vi "Main.vi"() -> ()   [LabVIEW 2026]
doc: "This Continuous Measurement sample project is based on the Queued Message Handler template.\n\nThe Event Handling Loop generates messages based on user interface actions.\n\nThe Message Handling Loop processes messages generated by the Event Handling Loop, or by other messages. There are also Acquisition and Logging message handling loop subVIs, and a chart updating loop."
uses:
  controls/UI State.ctl
  controls/UI Data.ctl
  Settings/Settings.ctl
  Acquisition/Hardware Configuration.ctl
  Acquisition/Signal Type.ctl
  Logging/Logging Configuration.ctl
  support/Message Queue/Enqueue Message (Single).vi
  support/Message Queue/Enqueue Message (Array).vi
  <vilib>/Utility/error.llb/Error Cluster From Error Code.vi
  <vilib>/ErrorRing/Error Ring.xnode
  Acquisition/Acquisition.lvlib
  Logging/Logging.lvlib
  Settings/Settings.lvlib
  support/User Event - Stop/User Event - Stop.lvlib
  support/Message Queue/Message Queue.lvlib
  Settings/Settings Dialog.vi
panel:
  out "Hardware Configuration.HW Refnum <Replace Me>":string
  out "Hardware Configuration.Signal Type <Replace Me>":T1
  out "Data":waveform(dbl)[](graph)
  in  "Settings":bool
  in  "Start":bool
  in  "Stop":bool
  out "Status":string
  in  "Exit":bool
  # "Continuous Measurement Data Logger"
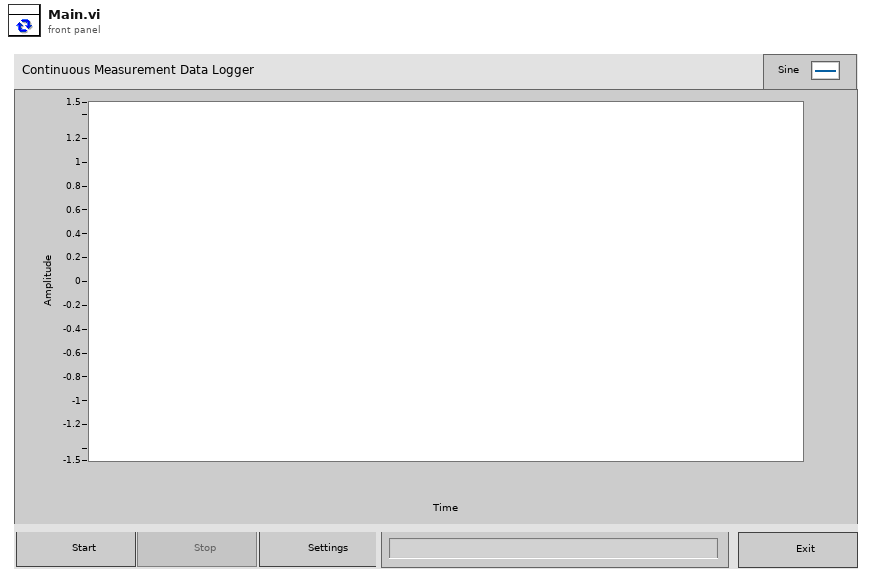
[diagram p1: front panel]
types:
  T1 = typedef "Acquisition.lvlib/Signal Type.ctl" = enum16{"Sine Wave", "Square with Noise"}
  T2 = typedef "UI State.ctl" = enum16{"Idle", "Acquiring and Logging", "Waiting for Exit", "Waiting for Exit (Acq Stopped)", "Waiting for Exit (Log Stopped)", "Waiting for Stop", "Waiting for Stop (Acq Stopped)", "Waiting for Stop (Log Stopped)"}
  T3 = typedef "UI Data.ctl" = cluster{"Start Ref":refnum<vi>, "Stop Ref":refnum<vi>, "Settings Ref":refnum<vi>, "Exit Ref":refnum<vi>, "Status Ref":refnum<vi>, "Data Ref":refnum<vi>}
  T4 = typedef "Settings.lvlib/Settings.ctl" = cluster{"Hardware Configuration":T5, "Logging Configuration":T6}
  T5 = typedef "Acquisition.lvlib/Hardware Configuration.ctl" = cluster{"HW Refnum <Replace Me>":string, "Signal Type <Replace Me>":T1}
  T6 = typedef "Logging.lvlib/Logging Configuration.ctl" = cluster{"Log File Base Path":path, "TDMS File Reference":refnum<k34>}
  T7 = typedef "Message Queue.lvlib/All Message Queues.ctl" = cluster{"UI":refnum<queue>, "Acquisition":refnum<queue>, "Logging":refnum<queue>}
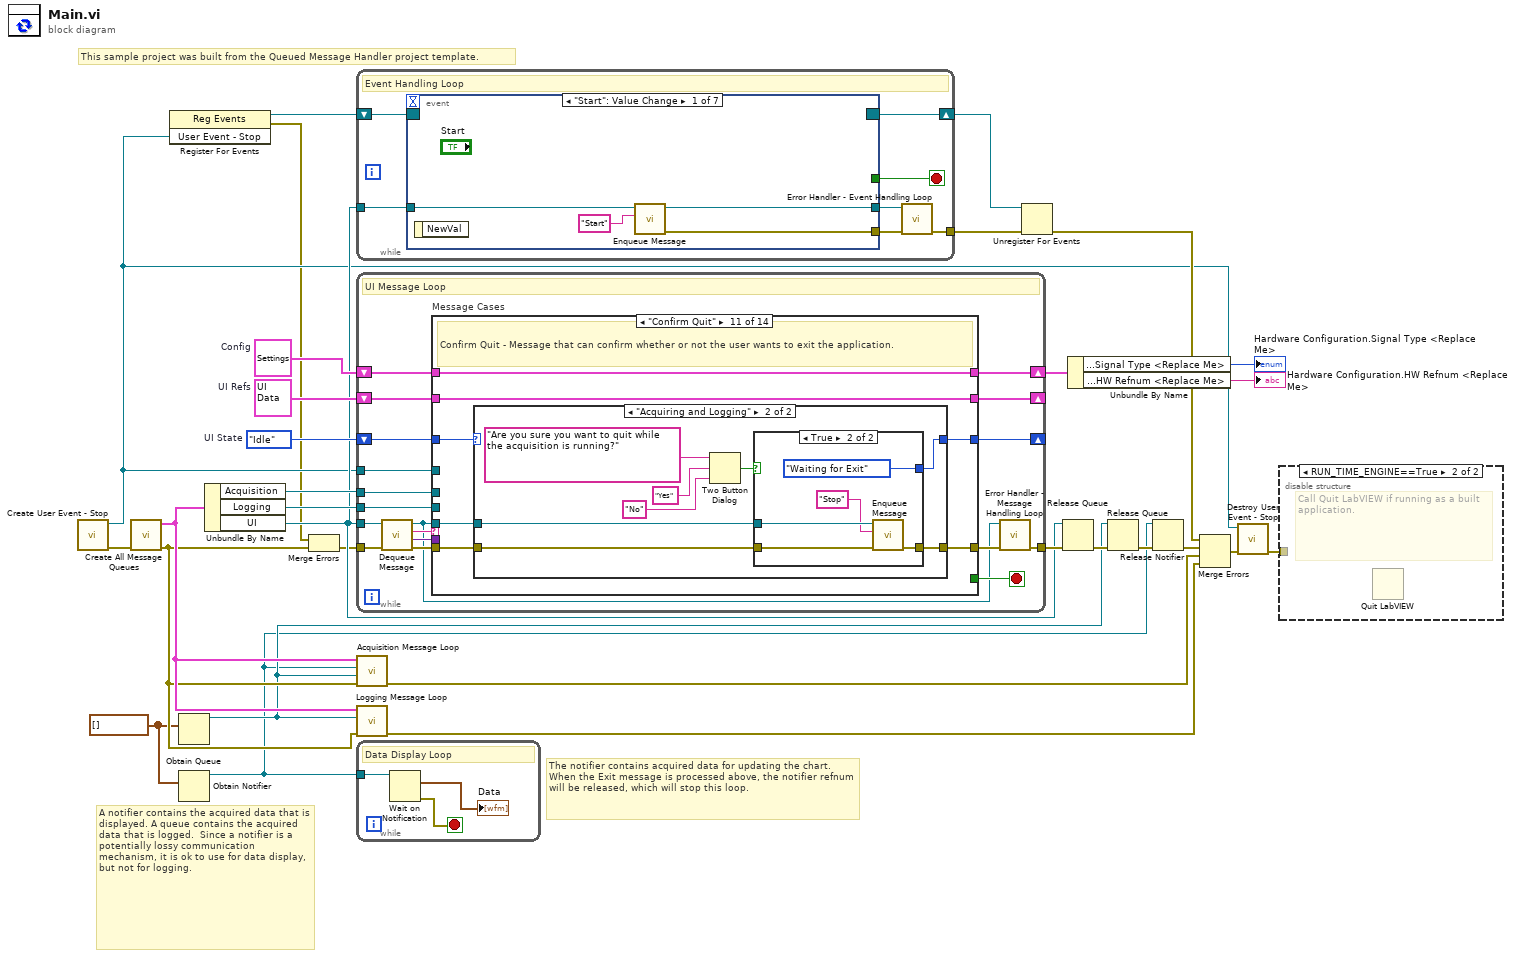
[diagram p0: block diagram]
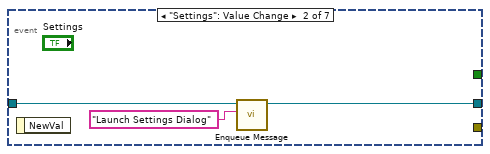
[diagram p3: hidden frame]
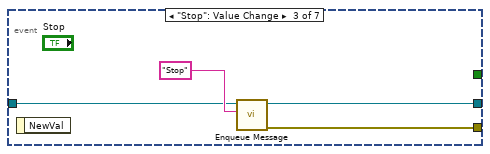
[diagram p4: hidden frame]
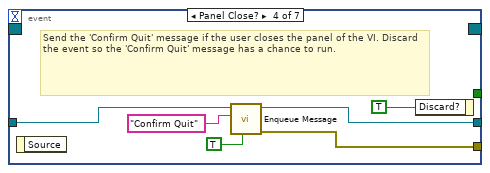
[diagram p5: hidden frame]
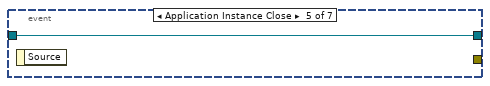
[diagram p6: hidden frame]
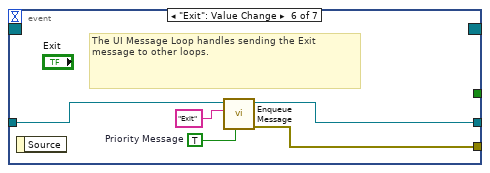
[diagram p7: hidden frame]
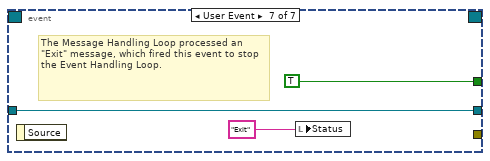
[diagram p8: hidden frame]
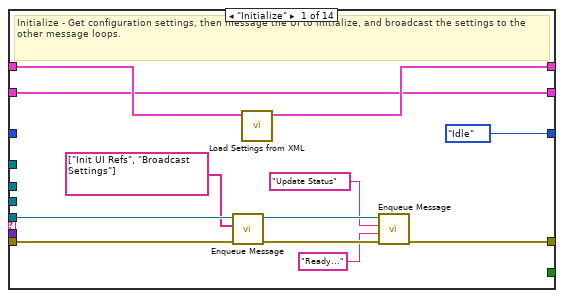
[diagram p9: hidden frame]
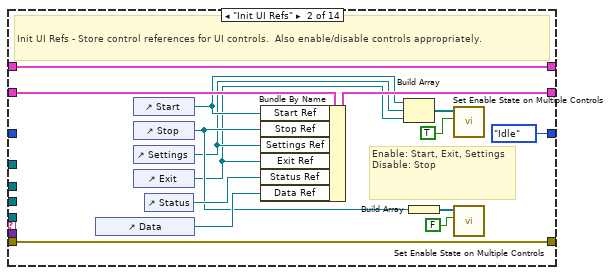
[diagram p10: hidden frame]
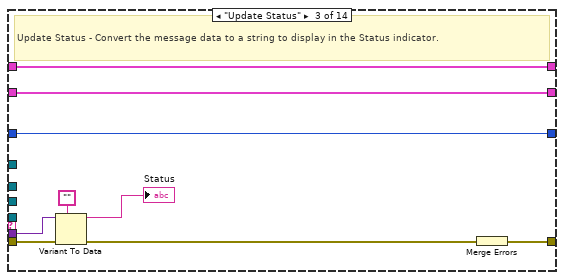
[diagram p11: hidden frame]
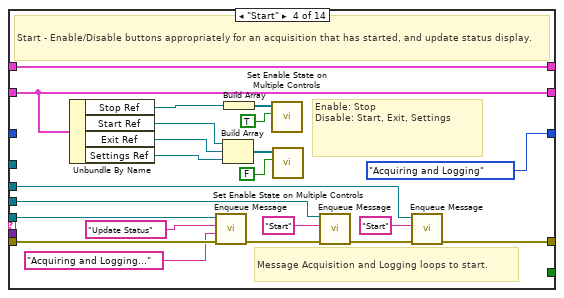
[diagram p12: hidden frame]
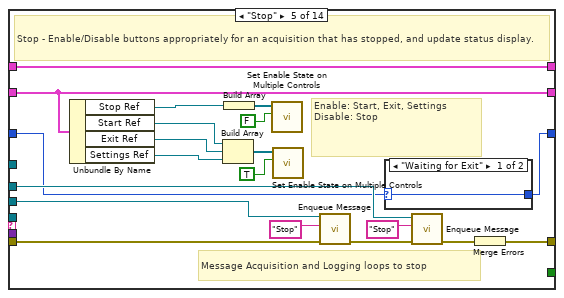
[diagram p13: hidden frame]
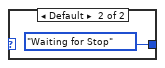
[diagram p14: hidden frame]
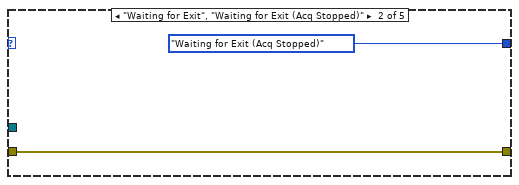
[diagram p16: hidden frame]
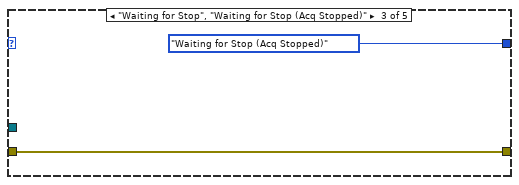
[diagram p17: hidden frame]
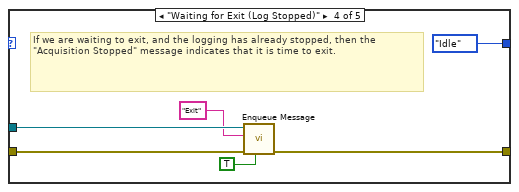
[diagram p18: hidden frame]
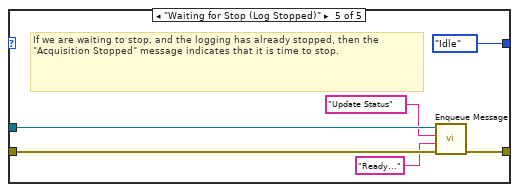
[diagram p19: hidden frame]
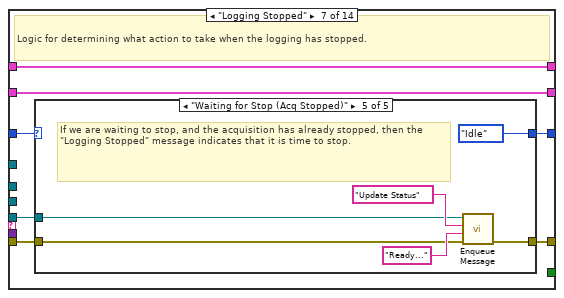
[diagram p20: hidden frame]
diagram:
  w17 = UI_State."Idle"  # UI State
  w8 = waveform(dbl)[] []
  w20 = T3 {"Start Ref"=refnum, "Stop Ref"=refnum, "Settings Ref"=refnum, "Exit Ref"=refnum, "Status Ref"=refnum, "Data Ref"=refnum}  # UI Refs
  w23 = T4 {"Hardware Configuration"={"HW Refnum <Replace Me>"="", "Signal Type <Replace Me>"=enum."Sine Wave"}, "Logging Configuration"={"Log File Base Path"=path "", "TDMS File Reference"=refnum}}  # Config
  # "This sample project was built from the Queued Message Handler project template."
  # "A notifier contains the acquired data that is displayed. A queue contains the acquired data that is logged.  Since a notifier is a potentially lossy communication mechanism, it is ok to use for data display, but not for logging."
  # "The notifier contains acquired data for updating the chart. When the Exit message is processed above, the notifier refnum will be released, which will stop this loop."
  n1 = call "Create User Event - Stop.vi"() -> ("error out"=w27:errorcluster, "User Event - Stop"=w6:refnum<user-event>)  [unwired: 10 in]
  n2 = call "Create All Message Queues.vi"("error in (no error)"=w27) -> ("error out"=w24:errorcluster, "Message Queues out"=w26:T7)  [unwired: 9 in]
  n3 = register-events(w6) -> (reference out=w7:refnum<event-registration>, error out=w4:errorcluster)  [unwired: 2 in]
  n4 = Obtain Queue(element data type=w8) -> (queue out=w10:refnum<queue>)  [unwired: 4 in, 2 out]
  n5 = Obtain Notifier(notification data type=w8) -> (notifier out=w9:refnum<notifier>)  [unwired: 3 in, 2 out]
  n6 = Unbundle By Name(w26) -> ("Acquisition"=w19:refnum<queue>, "Logging"=w18:refnum<queue>, "UI"=w15:refnum<queue>)
  n7 = Merge Errors(w4, w24) -> (w5:errorcluster)
  n8 = while {
    tunnel: w15 -> [w36]
    tunnel: [w33] -> w29
    shift-right: [w35] -> w21
    shift-left: w7 -> [w37]
    stop <- w34 stop-if-true
    # "Event Handling Loop"
    n9 = event shown="[0] \"Start\": Value Change" {
      selector: w37 -> [_ _ _ _ _ _ _]
      dyn-events: [_ _ _ _ _ _ _] -> w35
      timeout: _ -> [_ _ _ _ _ _ _]
      tunnel: [_ _ _ _ _ _ TRUE ("Discard?")] -> w34
      tunnel: w36 -> [w41 w43 w47 w52 w55 w57 w61]
      tunnel: [w39 _ w46 w50 _ w60 _] -> w32
      tunnel: [w38 w42 w45 w51 w55 w56 w61] -> w31
      event "Start": Value Change {
        n10 = event-data() -> ()  [unwired: 1 in, 1 out]
        n11 = call-poly "Enqueue Message.vi"("Message"="Start", "Message Queue"=w41) -> ("error out"=w39:errorcluster, "dup Message Queue"=w38:refnum<queue>)  [unwired: 8 in]
      }
      event "Settings": Value Change {
        n12 = event-data() -> ()  [unwired: 1 in, 1 out]
        n13 = call-poly "Enqueue Message.vi"("Message"="Launch Settings Dialog", "Message Queue"=w43) -> ("dup Message Queue"=w42:refnum<queue>)  [unwired: 8 in, 1 out]
      }
      event "Stop": Value Change {
        n14 = event-data() -> ()  [unwired: 1 in, 1 out]
        n15 = call-poly "Enqueue Message.vi"("Message"="Stop", "Message Queue"=w47) -> ("error out"=w46:errorcluster, "dup Message Queue"=w45:refnum<queue>)  [unwired: 8 in]
      }
      event Panel Close? {
        # "Send the 'Confirm Quit' message if the user closes the panel of the VI. Discard the event so the 'Confirm Quit' message has a chance to run."
        n16 = event-data() -> ()  [unwired: 1 in, 1 out]
        n17 = call-poly "Enqueue Message.vi"("Priority Message? (F)"=TRUE, "Message"="Confirm Quit", "Message Queue"=w52) -> ("error out"=w50:errorcluster, "dup Message Queue"=w51:refnum<queue>)  [unwired: 7 in]
        n18 = event-data("Discard?"=TRUE) -> ()  [unwired: 1 in, 1 out]
      }
      event Application Instance Close {
        n19 = event-data() -> ()  [unwired: 1 in, 1 out]
      }
      event "Exit": Value Change {
        w58 = TRUE  # Priority Message
        # "The UI Message Loop handles sending the Exit message to other loops."
        n20 = event-data() -> ()  [unwired: 1 in, 1 out]
        n21 = call-poly "Enqueue Message.vi"("Priority Message? (F)"=w58, "Message"="Exit", "Message Queue"=w57) -> ("error out"=w60:errorcluster, "dup Message Queue"=w56:refnum<queue>)  [unwired: 7 in]
      }
      event User Event {
        # "The Message Handling Loop processed an \"Exit\" message, which fired this event to stop the Event Handling Loop."
        n22 = event-data() -> ()  [unwired: 1 in, 1 out]
        n23 = local write "Status"("Exit" ("Exit String")) -> ()
      }
    }
    n24 = call "Error Handler - Event Handling Loop.vi"("error in (no error)"=w32, "Message Queue"=w31) -> ("dup error in"=w33:errorcluster)  [unwired: 8 in, 1 out]
  }
  n25 = while {
    tunnel: w15 -> [w75]
    tunnel: w6 -> [w80]
    shift-right: [w74] -> w3
    shift-left: w23 -> [w73]
    shift-right: [w71] -> _
    shift-left: w20 -> [w72]
    tunnel: w19 -> [w70]
    tunnel: w18 -> [w69]
    shift-right: [w64] -> _
    shift-left: w17 -> [w65]
    tunnel: w5 -> [w79]
    tunnel: [w68] -> w30
    stop <- w81 stop-if-true
    # "UI Message Loop"
    n26 = call "Dequeue Message.vi"("error in (no error)"=w79, "Message Queue"=w75) -> ("error out"=w78:errorcluster, "Message Data"=w76:variant, "Message"=w77:string, "dup Message Queue"=w66:refnum<queue>)  [unwired: 6 in]
    n27 = case "Message Cases" shown="\"Confirm Quit\"" w77 {
      selector: w77 -> [_ _ _ _ _ _ _ _ _ _ _ _ _ w297]
      tunnel: w66 -> [w85 _ _ w139 _ w164 w189 _ w229 _ w250 _ _ _]
      tunnel: w78 -> [w84 w108 w116 w138 w158 w165 w190 w217 w231 w238 w249 w278 w295 _]
      tunnel: [w89 w108 w117 w121 w159 w162 w187 w223 w224 w241 w248 w288 w294 w296] -> w67
      tunnel: [_ _ _ _ _ _ _ _ _ _ _ TRUE _ _] -> w81
      tunnel: w76 -> [_ _ w115 _ _ _ _ _ _ w242 _ w276 _ _]
      tunnel: w80 -> [_ _ _ _ _ _ _ _ _ _ _ w289 _ _]
      tunnel: [w92 w107 w111 w137 w157 w168 w193 w221 w228 w246 w253 w287 w293 w300] -> w74
      tunnel: w73 -> [w93 w107 w111 w137 w157 w168 w193 w221 w232 w246 w253 w287 w293 w300]
      tunnel: w72 -> [w86 w106 w110 w134 w156 w167 w192 w215 w226 w245 w252 w286 w292 w299]
      tunnel: [w86 w103 w110 w134 w156 w167 w192 w215 w226 w245 w252 w286 w292 w299] -> w71
      tunnel: w70 -> [_ _ _ w120 w143 _ _ w214 _ _ _ w285 _ _]
      tunnel: w69 -> [_ _ _ w123 w146 _ _ w213 _ _ _ w284 _ _]
      tunnel: w65 -> [_ _ w109 _ w140 w166 w191 w212 w225 w240 w251 _ w291 w298]
      tunnel: [UI_State."Idle" ("UI State") UI_State."Idle" ("UI State") w109 UI_State."Acquiring and Logging" ("UI State") w141 w163 w188 w212 w225 w240 w247 UI_State."Idle" ("UI State") w291 w298] -> w64
      frame "Initialize" {
        # "Initialize - Get configuration settings, then message the UI to initialize, and broadcast the settings to the other message loops."
        n28 = call-poly "Enqueue Message.vi"("error in (no error)"=w84, "Message Array"=string[] ["Init UI Refs", "Broadcast Settings"], "Message Queue"=w85) -> ("error out"=w91:errorcluster, "dup Message Queue"=w90:refnum<queue>)  [unwired: 7 in]
        n29 = call "Load Settings from XML.vi"("Settings in"=w93) -> ("Settings out"=w92:T4)  [unwired: 9 in, 1 out]
        n30 = call-poly "Enqueue Message.vi"("error in (no error)"=w91, "Message Data"="Ready..." ("Ready..."), "Message"="Update Status", "Message Queue"=w90) -> ("error out"=w89:errorcluster)  [unwired: 6 in, 1 out]
      }
      frame "Init UI Refs" {
        # "Enable: Start, Exit, Settings\nDisable: Stop"
        # "Init UI Refs - Store control references for UI controls.  Also enable/disable controls appropriately."
        n31 = control-ref of="Data"() -> (w104:refnum<vi>)
        n32 = control-ref of="Start"() -> (w97:refnum<vi>)
        n33 = control-ref of="Stop"() -> (w98:refnum<vi>)
        n34 = control-ref of="Settings"() -> (w96:refnum<vi>)
        n35 = control-ref of="Exit"() -> (w95:refnum<vi>)
        n36 = control-ref of="Status"() -> (w105:refnum<vi>)
        n37 = Bundle By Name(cluster=w106, "Start Ref"=w97, "Stop Ref"=w98, "Settings Ref"=w96, "Exit Ref"=w95, "Status Ref"=w105, "Data Ref"=w104) -> (w103:T3)
        n38 = Build Array(w97, w96, w95) -> (w101:refnum<vi>[])
        n39 = Build Array(w98) -> (w100:refnum<vi>[])
        n40 = call "Set Enable State on Multiple Controls.vi"("Enable?"=TRUE, "Controls"=w101) -> ()  [unwired: 10 in]
        n41 = call "Set Enable State on Multiple Controls.vi"("Enable?"=FALSE, "Controls"=w100) -> ()  [unwired: 10 in]
      }
      frame "Update Status" {
        # "Update Status - Convert the message data to a string to display in the Status indicator."
        n42 = Variant To Data(error in=w116, type="", Variant=w115) -> (data=→"Status":string, error out=w113:errorcluster)
        n43 = Merge Errors(w113) -> (w117:errorcluster)
      }
      frame "Start" {
        # "Message Acquisition and Logging loops to start."
        # "Enable: Stop\nDisable: Start, Exit, Settings"
        # "Start - Enable/Disable buttons appropriately for an acquisition that has started, and update status display."
        n44 = Unbundle By Name(w134) -> ("Stop Ref"=w129:refnum<vi>, "Start Ref"=w128:refnum<vi>, "Exit Ref"=w127:refnum<vi>, "Settings Ref"=w126:refnum<vi>)
        n45 = call-poly "Enqueue Message.vi"("error in (no error)"=w138, "Message Data"="Acquiring and Logging..." ("Acquiring and Logging..."), "Message"="Update Status", "Message Queue"=w139) -> ("error out"=w125:errorcluster)  [unwired: 6 in, 1 out]
        n46 = Build Array(w128, w127, w126) -> (w132:refnum<vi>[])
        n47 = Build Array(w129) -> (w131:refnum<vi>[])
        n48 = call "Set Enable State on Multiple Controls.vi"("Enable?"=TRUE, "Controls"=w131) -> ()  [unwired: 10 in]
        n49 = call "Set Enable State on Multiple Controls.vi"("Enable?"=FALSE, "Controls"=w132) -> ()  [unwired: 10 in]
        n50 = call-poly "Enqueue Message.vi"("error in (no error)"=w125, "Message"="Start", "Message Queue"=w123) -> ("error out"=w122:errorcluster)  [unwired: 7 in, 1 out]
        n51 = call-poly "Enqueue Message.vi"("error in (no error)"=w122, "Message"="Start", "Message Queue"=w120) -> ("error out"=w121:errorcluster)  [unwired: 7 in, 1 out]
      }
      frame "Stop" {
        # "Message Acquisition and Logging loops to stop"
        # "Enable: Start, Exit, Settings\nDisable: Stop"
        # "Stop - Enable/Disable buttons appropriately for an acquisition that has stopped, and update status display."
        n52 = Unbundle By Name(w156) -> ("Stop Ref"=w151:refnum<vi>, "Start Ref"=w150:refnum<vi>, "Exit Ref"=w149:refnum<vi>, "Settings Ref"=w148:refnum<vi>)
        n53 = Build Array(w150, w149, w148) -> (w154:refnum<vi>[])
        n54 = Build Array(w151) -> (w153:refnum<vi>[])
        n55 = call "Set Enable State on Multiple Controls.vi"("Enable?"=FALSE, "Controls"=w153) -> ()  [unwired: 10 in]
        n56 = call "Set Enable State on Multiple Controls.vi"("Enable?"=TRUE, "Controls"=w154) -> ()  [unwired: 10 in]
        n57 = call-poly "Enqueue Message.vi"("error in (no error)"=w158, "Message"="Stop", "Message Queue"=w146) -> ("error out"=w145:errorcluster)  [unwired: 7 in, 1 out]
        n58 = case shown="\"Waiting for Exit\"" w140 {
          selector: w140 -> [w160 _]
          tunnel: [w160 UI_State."Waiting for Stop" ("UI State")] -> w141
          frame "Waiting for Exit" {
          }
          frame Default {
          }
        }
        n59 = call-poly "Enqueue Message.vi"("error in (no error)"=w145, "Message"="Stop", "Message Queue"=w143) -> ("error out"=w144:errorcluster)  [unwired: 7 in, 1 out]
        n60 = Merge Errors(w144) -> (w159:errorcluster)
      }
      frame "Acquisition Stopped" {
        # "Logic for determining what action to take when the acquisition has stopped."
        n61 = case shown="Default" w166 {
          selector: w166 -> [w170 _ _ _ _]
          tunnel: w165 -> [w169 w172 w174 w180 w186]
          tunnel: w164 -> [_ _ _ w178 w183]
          tunnel: [w170 UI_State."Waiting for Exit (Acq Stopped)" ("UI State") UI_State."Waiting for Stop (Acq Stopped)" ("UI State") UI_State."Idle" ("UI State") UI_State."Idle" ("UI State")] -> w163
          tunnel: [w169 w172 w174 w179 w184] -> w162
          frame Default {
          }
          frame "Waiting for Exit", "Waiting for Exit (Acq Stopped)" {
          }
          frame "Waiting for Stop", "Waiting for Stop (Acq Stopped)" {
          }
          frame "Waiting for Exit (Log Stopped)" {
            # "If we are waiting to exit, and the logging has already stopped, then the \"Acquisition Stopped\" message indicates that it is time to exit."
            n62 = call-poly "Enqueue Message.vi"("Priority Message? (F)"=TRUE, "error in (no error)"=w180, "Message"="Exit", "Message Queue"=w178) -> ("error out"=w179:errorcluster)  [unwired: 6 in, 1 out]
          }
          frame "Waiting for Stop (Log Stopped)" {
            # "If we are waiting to stop, and the logging has already stopped, then the \"Acquisition Stopped\" message indicates that it is time to stop."
            n63 = call-poly "Enqueue Message.vi"("error in (no error)"=w186, "Message Data"="Ready..." ("Ready..."), "Message"="Update Status", "Message Queue"=w183) -> ("error out"=w184:errorcluster)  [unwired: 6 in, 1 out]
          }
        }
      }
      frame "Logging Stopped" {
        # "Logic for determining what action to take when the logging has stopped."
        n64 = case shown="\"Waiting for Stop (Acq Stopped)\"" w191 {
          selector: w191 -> [w195 _ _ _ _]
          tunnel: w190 -> [w194 w197 w199 w205 w208]
          tunnel: w189 -> [_ _ _ w203 w207]
          tunnel: [w195 UI_State."Waiting for Exit (Log Stopped)" ("UI State") UI_State."Waiting for Stop (Log Stopped)" ("UI State") UI_State."Idle" ("UI State") UI_State."Idle" ("UI State")] -> w188
          tunnel: [w194 w197 w199 w204 w206] -> w187
          frame Default {
          }
          frame "Waiting for Exit", "Waiting for Exit (Log Stopped)" {
          }
          frame "Waiting for Stop", "Waiting for Stop (Log Stopped)" {
          }
          frame "Waiting for Exit (Acq Stopped)" {
            # "If we are waiting to exit, and the acquisition has already stopped, then the \"Logging Stopped\" message indicates that it is time to exit."
            n65 = call-poly "Enqueue Message.vi"("Priority Message? (F)"=TRUE, "error in (no error)"=w205, "Message"="Exit", "Message Queue"=w203) -> ("error out"=w204:errorcluster)  [unwired: 6 in, 1 out]
          }
          frame "Waiting for Stop (Acq Stopped)" {
            # "If we are waiting to stop, and the acquisition has already stopped, then the \"Logging Stopped\" message indicates that it is time to stop."
            n66 = call-poly "Enqueue Message.vi"("error in (no error)"=w208, "Message Data"="Ready..." ("Ready..."), "Message"="Update Status", "Message Queue"=w207) -> ("error out"=w206:errorcluster)  [unwired: 6 in, 1 out]
          }
        }
      }
      frame "Broadcast settings" {
        w216 = "Update Settings" ("Message")
        # "Broadcast settings - Send the 'Update Settings' message to the Logging and Acquisition message loops."
        n67 = Unbundle By Name(w221) -> ("Hardware Configuration"=w220:T5, "Logging Configuration"=w219:T6)
        n68 = call-poly "Enqueue Message.vi"("Message Data"=w220, "Message"=w216, "Message Queue"=w214) -> ("error out"=w222:errorcluster)  [unwired: 7 in, 1 out]
        n69 = call-poly "Enqueue Message.vi"("error in (no error)"=w222, "Message Data"=w219, "Message"=w216, "Message Queue"=w213) -> ("error out"=w218:errorcluster)  [unwired: 6 in, 1 out]
        n70 = Merge Errors(w218, w217) -> (w223:errorcluster)
      }
      frame "Launch Settings Dialog" {
        # "Launch Settings Dialog - Launch the Settings Dialog when the user clicks the 'Settings' button."
        n71 = call-by-ref "?"("error in (no error)"=w231, "Settings in"=w232) -> ("error out"=w227:errorcluster, "Cancelled?"=w230:bool, "Settings out"=w228:T4)  [unwired: 8 in, 3 out]
        n72 = case shown="False" w230 {
          tunnel: w229 -> [w236 _]
          tunnel: w227 -> [w235 w237]
          tunnel: [w234 w237] -> w224
          frame False {
            n73 = call-poly "Enqueue Message.vi"("error in (no error)"=w235, "Message"="Broadcast Settings", "Message Queue"=w236) -> ("error out"=w234:errorcluster)  [unwired: 7 in, 1 out]
          }
          frame True {
          }
        }
      }
      frame "Error" {
        # "Error - Display an error dialog. This message is sent by the \"Error Handler\" VIs at the end of other loops in this application."
        n74 = Variant To Data(error in=w238, type=errorcluster {"status"=FALSE, "code"=0, "source"=""} ("error constant"), Variant=w242) -> (data=w239:errorcluster, error out=w243:errorcluster)
        n75 = call <vilib>:"Simple Error Handler.vi"("error in (no error)"=w239) -> ()  [unwired: 4 in, 5 out]
        n76 = Merge Errors(w243) -> (w241:errorcluster)
      }
      frame "Confirm Quit" {
        # "Confirm Quit - Message that can confirm whether or not the user wants to exit the application."
        n77 = case shown="\"Acquiring and Logging\"" w251 {
          tunnel: w250 -> [w259 w263]
          tunnel: w249 -> [w258 w262]
          tunnel: [w257 w261] -> w248
          tunnel: [UI_State."Idle" ("UI State") w260] -> w247
          frame Default {
            # "If 'Confirm Quit' comes in while the system is idle, there is no need for a confirmation message."
            n78 = call-poly "Enqueue Message.vi"("Priority Message? (F)"=TRUE, "error in (no error)"=w258, "Message"="Exit", "Message Queue"=w259) -> ("error out"=w257:errorcluster)  [unwired: 6 in, 1 out]
          }
          frame "Acquiring and Logging" {
            n79 = Two Button Dialog(message="Are you sure you want to quit while the acquisition is running?" ("Confirm Quit Message"), 1:"No" ("No"), 2:"Yes" ("Yes")) -> (T button?=w264:bool)
            n80 = case shown="True" w264 {
              tunnel: w263 -> [_ w273]
              tunnel: w262 -> [w269 w274]
              tunnel: [w269 w272] -> w261
              tunnel: [UI_State."Acquiring and Logging" ("UI State") UI_State."Waiting for Exit" ("UI State")] -> w260
              frame False {
                # "User did not want to quit."
              }
              frame True {
                n81 = call-poly "Enqueue Message.vi"("error in (no error)"=w274, "Message"="Stop", "Message Queue"=w273) -> ("error out"=w272:errorcluster)  [unwired: 7 in, 1 out]
              }
            }
          }
        }
      }
      frame "Exit" {
        w280 = TRUE ("Priority Message? (F)")
        w281 = "Exit" ("Message")
        # "Popup an error dialog if 'Exit' was called as a result of an error."
        # "Stop the VI"
        # "Exit - Send Exit messages to the Acquisition and Logging loops, and fire the user event to stop the Event Handling Loop."
        n82 = Variant To Data(type=errorcluster {"status"=FALSE, "code"=0, "source"=""} ("error constant"), Variant=w276) -> (data=w275:errorcluster)  [unwired: 1 in, 1 out]
        n83 = call <vilib>:"Simple Error Handler.vi"("error in (no error)"=w275) -> ()  [unwired: 4 in, 5 out]
        n84 = call-poly "Enqueue Message.vi"("Priority Message? (F)"=w280, "error in (no error)"=w278, "Message"=w281, "Message Queue"=w285) -> ("error out"=w282:errorcluster)  [unwired: 6 in, 1 out]
        n85 = call-poly "Enqueue Message.vi"("Priority Message? (F)"=w280, "error in (no error)"=w282, "Message"=w281, "Message Queue"=w284) -> ("error out"=w279:errorcluster)  [unwired: 6 in, 1 out]
        n86 = call "Fire User Event - Stop.vi"("error in (no error)"=w279, "User Event - Stop"=w289) -> ("error out"=w288:errorcluster)  [unwired: 9 in]
      }
      frame "---Copy This Frame---" {
        # "Duplicate this frame when creating new messages.  Change this comment in the duplicated frame to describe this message."
        n87 = Merge Errors(w295) -> (w294:errorcluster)
      }
      frame Default {
        # "'Default' case only runs if there is a message that isn't defined in any of the other cases.  Output a programming error."
        n88 = xnode "Error Ring"("parameter 0"=w297) -> ("error out"=w296:errorcluster)
      }
    }
    n89 = call "Error Handler - Message Handling Loop.vi"("error in (no error)"=w67, "Message Queue"=w66) -> ("dup error in"=w68:errorcluster)  [unwired: 8 in, 1 out]
  }
  n90 = call "Acquisition Message Loop.vi"("error in (no error)"=w24, "Data Queue"=w10, "Data Notifier"=w9, "Message Queues"=w26) -> ("error out"=w28:errorcluster)  [unwired: 7 in]
  n91 = call "Logging Message Loop.vi"("error in (no error)"=w24, "Data Queue"=w10, "Message Queues"=w26) -> ("error out"=w25:errorcluster)  [unwired: 8 in]
  n92 = while "Data Display Loop" {
    tunnel: w9 -> [w310]
    stop <- w308 stop-if-true
    # "Data Display Loop"
    n93 = Wait on Notification(notifier=w310) -> (notification=→"Data":waveform(dbl)[], error out=w308:errorcluster)  [unwired: 3 in, 2 out]
  }
  n94 = Unregister For Events(event registration refnum=w21, error in=w29) -> (error out=w22:errorcluster)
  n95 = Release Queue(queue=w15, error in (no error)=w30) -> (error out=w13:errorcluster)  [unwired: 1 in, 2 out]
  n96 = Unbundle By Name(w3) -> ("Hardware Configuration.Signal Type <Replace Me>"=→"Hardware Configuration.Signal Type <Replace Me>":T1, "Hardware Configuration.HW Refnum <Replace Me>"=→"Hardware Configuration.HW Refnum <Replace Me>":string)
  n97 = Release Queue(queue=w10, error in (no error)=w13) -> (error out=w12:errorcluster)  [unwired: 1 in, 2 out]
  n98 = Release Notifier(notifier=w9, error in (no error)=w12) -> (error out=w11:errorcluster)  [unwired: 1 in, 2 out]
  n99 = Merge Errors(w22, w11, w28, w25) -> (w16:errorcluster)
  n100 = call "Destroy User Event - Stop.vi"("error in (no error)"=w16, "User Event - Stop"=w6) -> ("error out"=w14:errorcluster)  [unwired: 9 in]
  n101 = disable-structure shown="RUN_TIME_ENGINE==True" {
    disable-tunnel: w14 -> [_ _]
    frame condition #0 (active) {
    }
    frame condition #1 {
      # "Call Quit LabVIEW if running as a built application."
      n102 = Quit LabVIEW() -> ()  [unwired: 1 in]
    }
  }
